vi "Create H2H Flag Array.vi"(10 "H2H Cutoff":i32=1, 11 "H2H Array":i32[][](array[numeric])) -> (3 "H2H Flag":bool[][](array[boolean]))   [LabVIEW 2013]
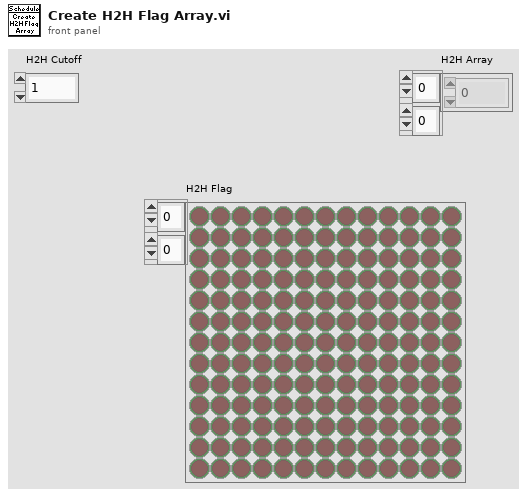
[diagram p1: front panel]
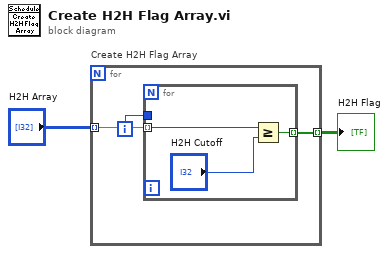
[diagram p0: block diagram]
diagram:
  n1 = for "Create H2H Flag Array" {
    tunnel: "H2H Array" -> [w5] mode=indexing
    tunnel: [w3] -> w2 mode=indexing
    i -> [w4]
    n2 = for {
      tunnel: w5 -> [w8] mode=indexing
      tunnel: w4 -> [_]
      tunnel: [w6] -> w3 mode=indexing
      n3 = Greater Or Equal?(x=w8, y="H2H Cutoff") -> (x >= y?=w6:bool)
    }
  }
  "H2H Flag" <- w2
